vi "Error Query.vi"(8 "error in (no error)":errorcluster, 11 "VISA resource name":refnum<visa-resource-name>) -> (0 "error out":errorcluster, 1 "Error Message":string, 2 "Error Code":i32[](array[numeric]), 3 "VISA resource name out":refnum<visa-resource-name>)   [LabVIEW 2018, in "Counter.lvlib" / "PICOTEST U62XXA series.lvlib"]
doc: "Queries the instrument for any errors in the instrument's error queue. It will continue to read errors until all errors have been read from the instrument. Any errors will be returned in the Error Code and Error Message Indicators as well as in the <B>error out</B> indicator.\n\n<B> Note:</B>\n\nThis VI is called automatically by most driver VIs so it is not usually necessary to call this in an application."
uses:
  PICOTEST U62XXA series.lvlib
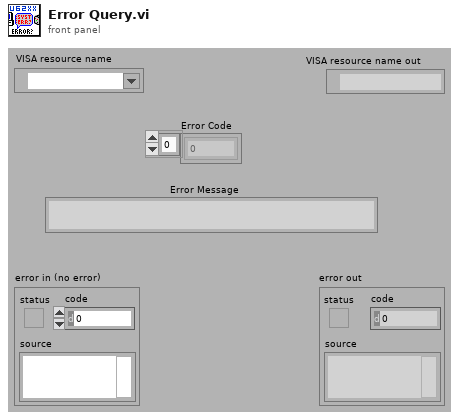
[diagram p1: front panel]
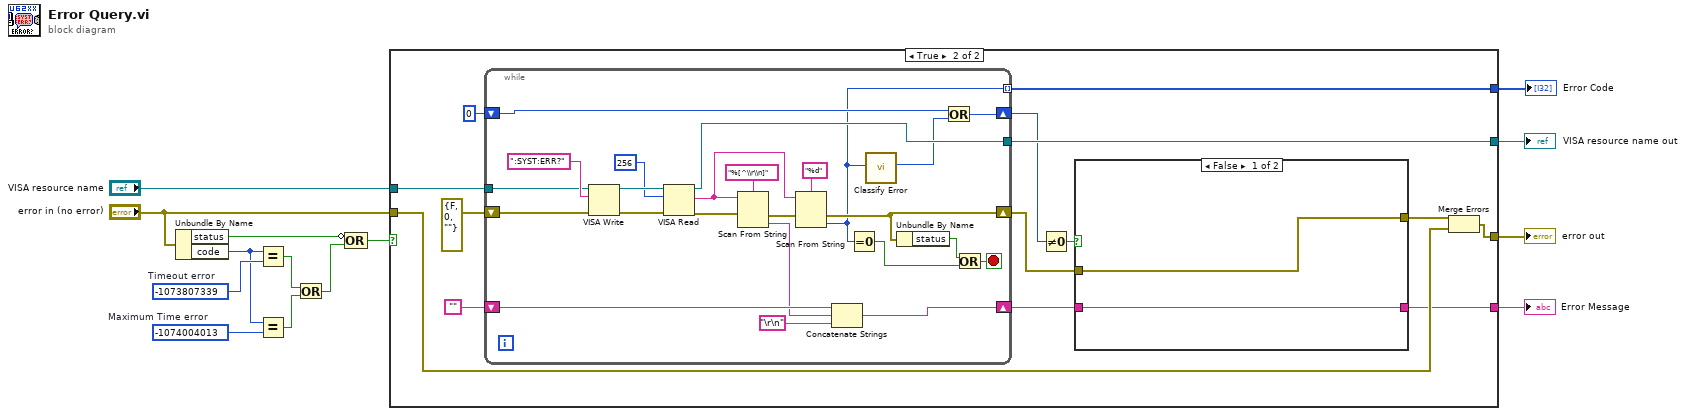
[diagram p0: block diagram]
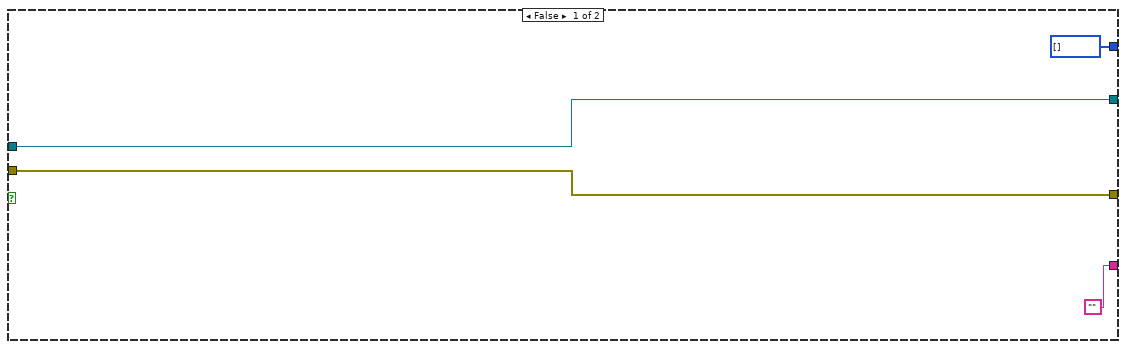
[diagram p2: hidden frame]
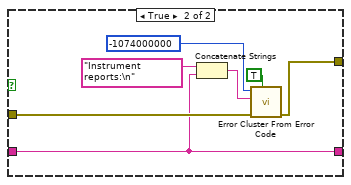
[diagram p3: hidden frame]
diagram:
  w5 = -1074004013  # Maximum Time error
  w10 = -1073807339  # Timeout error
  n1 = Unbundle By Name("error in (no error)") -> ("status"=w6:bool, "code"=w4:i32)
  n2 = Equal?(x=w4, y=w10) -> (x = y?=w2:bool)
  n3 = Equal?(x=w4, y=w5) -> (x = y?=w3:bool)
  n4 = Or(x=w2, y=w3) -> (x .or. y?=w1:bool)
  n5 = Compound Arithmetic op=OR(invert w6, w1) -> (w7:bool)
  n6 = case shown="True" w7 {
    tunnel: [w18 w32] -> w14
    tunnel: "VISA resource name" -> [w18 w31]
    tunnel: "error in (no error)" -> [w17 w26]
    tunnel: [w17 w30] -> w12
    tunnel: ["" w22] -> w9
    tunnel: [i32[] [] w27] -> w8
    frame False {
    }
    frame True {
      n7 = while {
        tunnel: [w65] -> w32
        tunnel: w31 -> [w42]
        shift-right: [w53] -> w23
        shift-left: "" -> [w56]
        shift-right: [w52] -> w24
        shift-left: errorcluster {"status"=FALSE, "code"=0, "source"=""} ("error in (no error)") -> [w43]
        tunnel: [w45] -> w27 mode=indexing
        shift-right: [w48] -> w19
        shift-left: 0 -> [w47]
        stop <- w59 stop-if-true
        n8 = VISA Write(VISA resource name=w42, write buffer=":SYST:ERR?", error in (no error)=w43) -> (VISA resource name out=w64:refnum<visa-resource-name>, error out=w62:errorcluster)  [unwired: 1 out]
        n9 = VISA Read(VISA resource name=w64, byte count=u32 256, error in (no error)=w62) -> (VISA resource name out=w65:refnum<visa-resource-name>, read buffer=w57:string, error out=w51:errorcluster)  [unwired: 1 out]
        n10 = Scan From String(format string="%[^\\r\\n]", input string=w57, error in=w51) -> (error out=w50:errorcluster, output 1=w54:string)  [unwired: 2 in, 2 out]
        n11 = Scan From String(format string="%d", input string=w57, error in=w50) -> (error out=w52:errorcluster, output 1=w45:i32)  [unwired: 2 in, 2 out]
        n12 = Concatenate Strings(w56, w54, "\r\n") -> (w53:string)
        n13 = Equal To 0?(x=w45) -> (x = 0?=w46:bool)
        n14 = call "Classify Error.vi"("Error Code"=w45) -> ("Error Classification"=w44:i32)  [unwired: 10 in]
        n15 = Unbundle By Name(w52) -> ("status"=w49:bool)
        n16 = Or(x=w47, y=w44) -> (x .or. y?=w48:i32)
        n17 = Or(x=w49, y=w46) -> (x .or. y?=w59:bool)
      }
      n18 = Not Equal To 0?(x=w19) -> (x != 0?=w20:bool)
      n19 = case shown="False" w20 {
        tunnel: [w34 w41] -> w29
        tunnel: w24 -> [w34 w36]
        tunnel: w23 -> [w33 w35]
        tunnel: [w33 w35] -> w22
        frame False {
        }
        frame True {
          n20 = Concatenate Strings("Instrument reports:\n" ("Source"), w35) -> (w37:string)
          n21 = call <vilib>:"Error Cluster From Error Code.vi"("show call chain? (False)"=TRUE, "error in (no error)"=w36, "error message (\"\")"=w37, "error code (0)"=-1074000000 ("Code")) -> ("error out"=w41:errorcluster)  [unwired: 5 in]
        }
      }
      n22 = Merge Errors(w29, w26) -> (w30:errorcluster)
    }
  }
  "VISA resource name out" <- w14
  "error out" <- w12
  "Error Message" <- w9
  "Error Code" <- w8
